vi "Update Status Bar Cycles.vi"(4 "Cycles":i32, 5 "Status Bar":refnum<vi>) -> (1 "Status Bar Out":refnum<vi>)   [LabVIEW 2011]
panel:
  out "error out":errorcluster
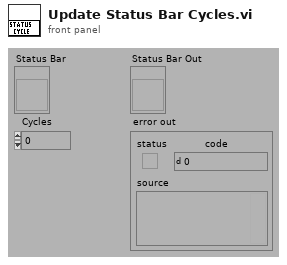
[diagram p1: front panel]
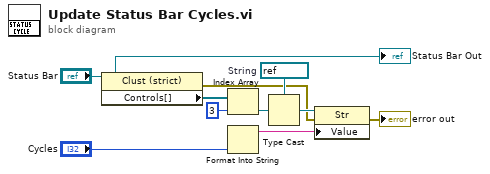
[diagram p0: block diagram]
diagram:
  w4 = refnum<vi> refnum  # String
  n1 = property class="Clust (strict)"(reference="Status Bar") -> (error out=w1:errorcluster, "Controls[]"=w6:refnum<vi>[])  [unwired: 1 in, 1 out]
  n2 = Index Array(array=w6, index=3) -> (element=w3:refnum<vi>)
  n3 = Format Into String("Cycles") -> (resulting string=w8:string)  [unwired: 3 in, 1 out]
  n4 = Type Cast(type=w4, x=w3) -> (*(type *) &x=w2:refnum<vi>)
  n5 = property class="Str"(reference=w2, error in=w1, "Value"=w8) -> (error out=→"error out":errorcluster)  [unwired: 1 out]
  "Status Bar Out" <- "Status Bar"
